vi "Init.vi"(3 "Container State":T3, 4 "Previous State":variant, 5 "Previous Version":T2) -> (2 "Current State":T1)   [LabVIEW 2020, in "Advanced Stimulus Options.xctl"]
uses:
  Advanced Stimulus Options.xctl
  State.ctl
  <vilib>/_xctls/Container State.ctl
  <vilib>/_xctls/Version.ctl
  State V1.ctl
  <vilib>/_xctls/XControlSupport.lvlib
panel:
  in  "Default Indicator State":T1
  in  "Default Control State":T1
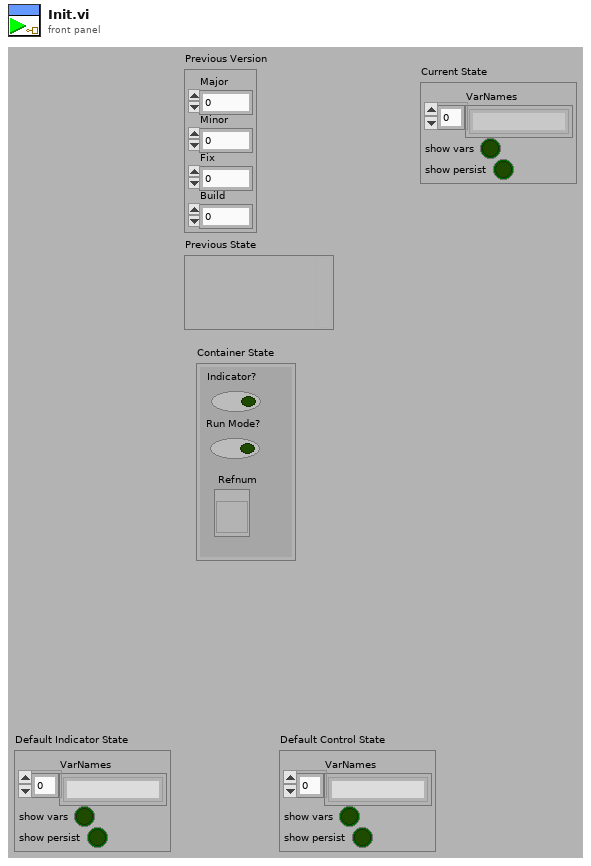
[diagram p1: front panel]
types:
  T1 = typedef "Advanced Stimulus Options.xctl/State.ctl" = cluster{"VarNames":string[], "show vars":bool, "show persist":bool}
  T2 = typedef "XControlSupport.lvlib/Version.ctl" = cluster{"Major":u16, "Minor":u16, "Fix":u16, "Build":u16}
  T3 = typedef "XControlSupport.lvlib/Container State.ctl" = cluster{"Indicator?":bool, "Run Mode?":bool, " Refnum":refnum<vi>}
  T4 = typedef "Advanced Stimulus Options.xctl/State V1.ctl" = cluster{"VarNames":string[], "show vars":bool}
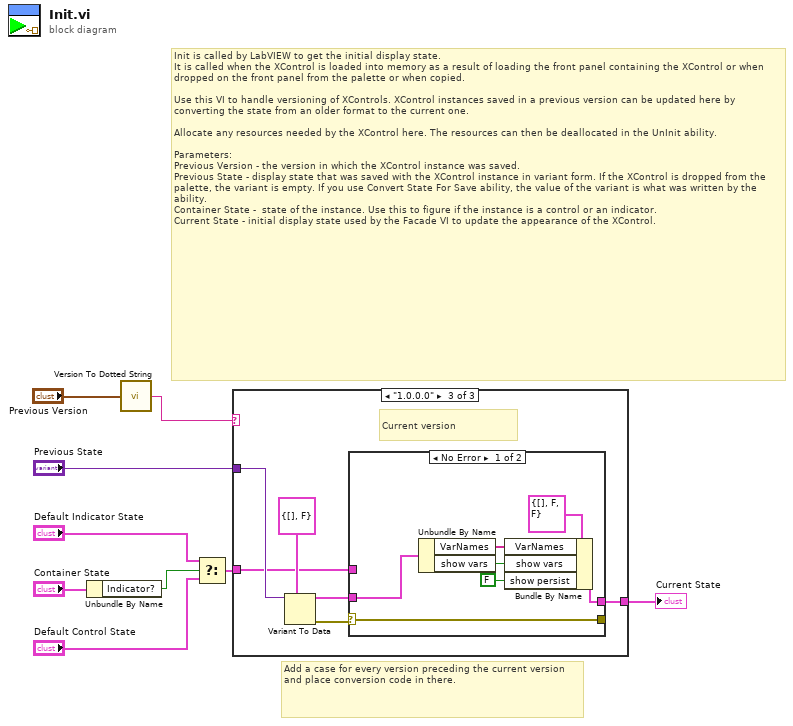
[diagram p0: block diagram]
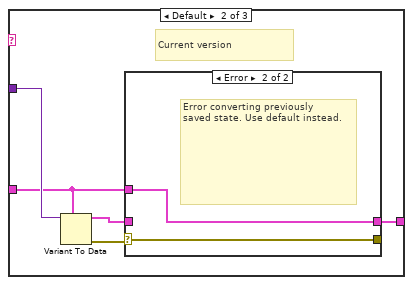
[diagram p3: hidden frame]
diagram:
  # "Add a case for every version preceding the current version and place conversion code in there."
  # "Init is called by LabVIEW to get the initial display state.\nIt is called when the XControl is loaded into memory as a result of loading the front panel containing the XControl or when dropped on the front panel from the palette or when copied.\n\nUse this VI to handle versioning of XControls. XControl instances saved in a previous version can be updated here by converting the state from an older format to the current one.\n\nAllocate any resources needed by the XControl here. The resources can then be deallocated in the UnInit ability.\n\nParameters:\nPrevious Version - the version in which the XControl instance was saved.\nPrevious State - display state that was saved with the XControl instance in variant form. If the XControl is dropped from the palette, the variant is empty. If you use Convert State For Save ability, the value of the variant is what was written by the ability. \nContainer State -  state of the instance. Use this to figure if the instance is a control or an indicator.\nCurrent State - initial display state used by the Facade VI to update the appearance of the XControl."
  n1 = Unbundle By Name("Container State") -> ("Indicator?"=w4:bool)
  n2 = call <vilib>:"Version To Dotted String.vi"("Version"="Previous Version") -> ("String Version"=w1:string)
  n3 = Select(t="Default Indicator State", s=w4, f="Default Control State") -> (s? t:f=w3:T1)
  n4 = case shown="\"1.0.0.0\"" w1 {
    tunnel: "Previous State" -> [_ w15 w25]
    tunnel: [w10 w11 w22] -> w8
    tunnel: w3 -> [w10 w12 w20]
    frame "0.0.0.0" {
      # "Just created, use default state"
    }
    frame Default {
      # "Current version"
      n5 = Variant To Data(type=w12, Variant=w15) -> (data=w13:T1, error out=w14:errorcluster)  [unwired: 1 in]
      n6 = case shown="Error" w14 {
        selector: w14 -> [w17 w18]
        tunnel: w13 -> [w16 _]
        tunnel: [w16 w19] -> w11
        tunnel: w12 -> [_ w19]
        tunnel: [w17 w18] -> _
        frame No Error {
        }
        frame Error {
          # "Error converting previously \nsaved state. Use default instead."
        }
      }
    }
    frame "1.0.0.0" {
      # "Current version"
      n7 = Variant To Data(type=T4 {"VarNames"=[], "show vars"=FALSE} ("State"), Variant=w25) -> (data=w23:T4, error out=w24:errorcluster)  [unwired: 1 in]
      n8 = case shown="No Error" w24 {
        selector: w24 -> [w27 w34]
        tunnel: w23 -> [w32 _]
        tunnel: [w26 w33] -> w22
        tunnel: [w27 w34] -> _
        tunnel: w20 -> [_ w33]
        frame No Error {
          n9 = Unbundle By Name(w32) -> ("VarNames"=w29:string[], "show vars"=w30:bool)
          n10 = Bundle By Name(cluster=T1 {"VarNames"=[], "show vars"=FALSE, "show persist"=FALSE} ("Current State"), "VarNames"=w29, "show vars"=w30, "show persist"=FALSE) -> (w26:T1)
        }
        frame Error {
          # "Error converting previously \nsaved state. Use default instead."
        }
      }
    }
  }
  "Current State" <- w8
